vi "clear.vi"(8 "error in (no error)":errorcluster, 11 "Map in":refnum<class "Map.lvclass">) -> (0 "error out":errorcluster, 3 "Map out":refnum<class "Map.lvclass">)   [LabVIEW 2010, in "Map.lvclass"]
doc: "This method deletes all elements from the map."
uses:
  Map.lvclass
  element_cluster.ctl
  Map.lvclass/Map.ctl
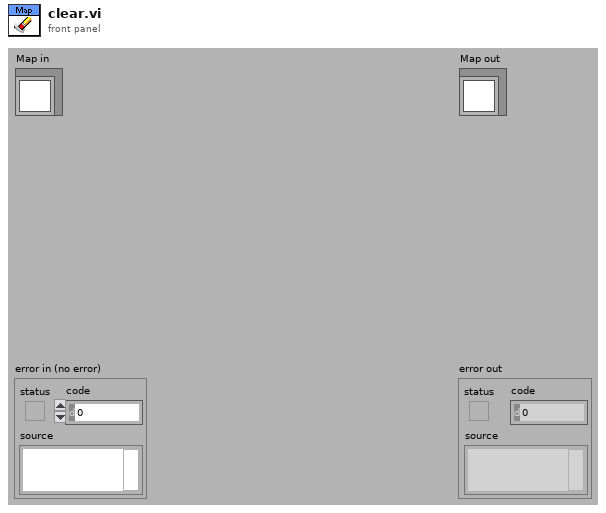
[diagram p1: front panel]
types:
  T1 = typedef "Map.lvclass/element_cluster.ctl" = cluster{"key":string, "value":variant}
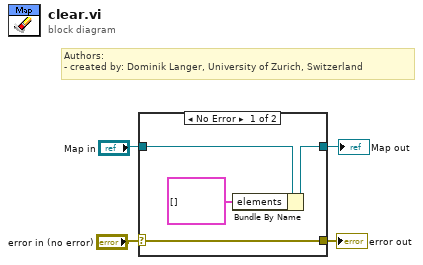
[diagram p0: block diagram]
diagram:
  # "Authors: \n- created by: Dominik Langer, University of Zurich, Switzerland"
  n1 = case shown="No Error" "error in (no error)" {
    selector: "error in (no error)" -> [w8 w10]
    tunnel: [w8 w10] -> w3
    tunnel: [w6 w9] -> w1
    tunnel: "Map in" -> [w7 w9]
    frame No Error {
      n2 = Bundle By Name(cluster=w7, "elements"=T1[] []) -> (w6:refnum<class "Map.lvclass">)
    }
    frame Error {
    }
  }
  "error out" <- w3
  "Map out" <- w1
